vi "SOMD.vi"(8 "Stopp":bool, 10 "SLOT":i32=100, 11 "USB":i32) -> ()   [LabVIEW 2020]
doc: "This VI provides a GUI for SOM-D modules. It implements an abstract module interface, where callers provide the only necessary and sufficient information for callee modules via the datafields USB, SLOT and Stopp. All module intern information are handled hidden by the module. Thereby, a caller must not \"know\" about such internals."
uses:
  <vilib>/Platform/TimedLoop/XDataNode/timing_clust.ctl
  <vilib>/Platform/TimedLoop/XDataNode/nitl_modes.ctl
  <vilib>/Platform/TimedLoop/XDataNode/wakeup.ctl
  <vilib>/platform/TimedLoop/XDataNode/XDataNode.xnode
  <vilib>/Platform/TimedLoop/XDataNode/XDNodeRunTimeDep.lvlib
panel:
  out "DisableBlend":string
  in  "Delayed Data":T1(array[cluster])
  in  "DelayedData[i]":cluster{"Delayed":bool, "ForcedUndelayed":bool}
  in  "SyncNow":bool
  out "SOMD Status":string
  in  "CombiDat 2":T2={"OutputCombi[i]"=[], "MaskedCombi[i]"=TRUE}
  in  "DelayDat 5":cluster{"CoarseDelay[i]":dbl, "FineDelay[i]":u8} {"CoarseDelay[i]" min=-999999.9 max=999999.9 step=1.0 format="%.1f"; "FineDelay[i]" max=63 step=1}
  in  "DelayDat 3":cluster{"CoarseDelay[i]":dbl, "FineDelay[i]":u8} {"CoarseDelay[i]" min=-999999.9 max=999999.9 step=1.0 format="%.1f"; "FineDelay[i]" max=63 step=1}
  in  "DelayDat 6":cluster{"CoarseDelay[i]":dbl, "FineDelay[i]":u8} {"CoarseDelay[i]" min=-999999.9 max=999999.9 step=1.0 format="%.1f"; "FineDelay[i]" max=63 step=1}
  in  "DelayDat 1":cluster{"CoarseDelay[i]":dbl, "FineDelay[i]":u8} {"CoarseDelay[i]" min=-999999.9 max=999999.9 step=1.0 format="%.1f"; "FineDelay[i]" max=63 step=1}
  in  "CombiDat 8":T2={"OutputCombi[i]"=[], "MaskedCombi[i]"=TRUE}
  in  "CombiDat 7":T2={"OutputCombi[i]"=[], "MaskedCombi[i]"=TRUE}
  in  "CombiDat 4":T2={"OutputCombi[i]"=[], "MaskedCombi[i]"=TRUE}
  out "FreqStable":bool caption="stable"
  out "FreqMeasTimer":u32
  out "ExtTriggrd":bool
  out "Trigger Frequency":u32 caption="Trig. Freq. [Hz]"
  in  "CombiDat 5":T2={"OutputCombi[i]"=[], "MaskedCombi[i]"=TRUE}
  in  "CombiDat 3":T2={"OutputCombi[i]"=[], "MaskedCombi[i]"=TRUE}
  in  "DelayDat 8":cluster{"CoarseDelay[i]":dbl, "FineDelay[i]":u8} {"CoarseDelay[i]" min=-999999.9 max=999999.9 step=1.0 format="%.1f"; "FineDelay[i]" max=63 step=1}
  in  "DelayDat 7":cluster{"CoarseDelay[i]":dbl, "FineDelay[i]":u8} {"CoarseDelay[i]" min=-999999.9 max=999999.9 step=1.0 format="%.1f"; "FineDelay[i]" max=63 step=1}
  in  "DelayDat 4":cluster{"CoarseDelay[i]":dbl, "FineDelay[i]":u8} {"CoarseDelay[i]" min=-999999.9 max=999999.9 step=1.0 format="%.1f"; "FineDelay[i]" max=63 step=1}
  in  "CombiDat 6":T2={"OutputCombi[i]"=[], "MaskedCombi[i]"=TRUE}
  in  "CombiDat 1":T2={"OutputCombi[i]"=[], "MaskedCombi[i]"=TRUE}
  in  "Delay Data":T3(array[cluster]) {"CoarseDelay[i]" min=-999999.9 max=999999.9 step=1.0 format="%.1f"; "FineDelay[i]" max=63 step=1}
  in  "DelayDat[i]":cluster{"CoarseDelay[i]":dbl, "FineDelay[i]":u8} {"CoarseDelay[i]" min=-999999.9 max=999999.9 step=1.0 format="%.1f"; "FineDelay[i]" max=63 step=1}
  in  "CombiDat[i]":T2={"OutputCombi[i]"=[], "MaskedCombi[i]"=TRUE}
  in  "Combi Data":T4(array[cluster])
  in  "OutputCombi[i]":bool[](array[boolean])
  in  "Coarse Delay":dbl[](array[numeric])=[1.0, 0.0, 2.0, 0.0, 0.0, 0.0, 0.0, 0.0] min=-999999.9 max=999999.9 format="%.1f"
  in  "Fine Delay":u8[](array[numeric])=[1, 0, 2, 0, 0, 0, 0, 0] max=63 step=1
  in  "BurstDat[i]":T5={"[i]"=1, "BurstLen[i]"=1, "SyncEna[i]"=TRUE, "OutpEna[i]"=TRUE, "Delayed[i]"=TRUE} {"BurstLen[i]" min=0 max=16777215 step=1}
  in  "Burst Data":T6(array[cluster]) {"BurstLen[i]" min=0 max=16777215 step=1}
  in  "AUX In Ctrl":u8(ring) items=["free running", "running if AUX IN is on High", "running if AUX IN is on Low", "disabled"]
  in  "AUX Out Ctrl":u8(ring) items=["disabled", "enabled"]
  in  "Synchronize":bool
  in  "Sync Enable":bool[](array[boolean])=[TRUE, FALSE, FALSE, TRUE, FALSE, FALSE, FALSE, FALSE]
  in  "Burst Out":bool[](array[boolean])=[TRUE, TRUE, FALSE, FALSE, TRUE, FALSE, FALSE, FALSE]
  in  "TriggerLevel [mV]":i32=421 caption="Trig. Level [mV]" min=-1200 max=1200 step=100 format="%5d"
  in  "Burst Length":i32[](array[numeric])=[1, 0, 2, 0, 0, 0, 0, 0]
  in  "Invert":bool=TRUE
  in  "Syncmask":u8
  in  "Presync":u8=4
  in  "Divider":u16=80 min=1 step=1
  in  "Base Osc./Trigger":i32(ring)=2 items=["rising  edge (ext.)", "falling edge (ext.)", "80.00 MHz (int. A)", "64.00 MHz (int. B)", "50.00 MHz (int. C)"]
  in  "DelayDat 2":cluster{"CoarseDelay[i]":dbl, "FineDelay[i]":u8} {"CoarseDelay[i]" min=-999999.9 max=999999.9 step=1.0 format="%.1f"; "FineDelay[i]" max=63 step=1}
  # "Idx   Burst Length       Sync Ena   Out Ena   Delayed"
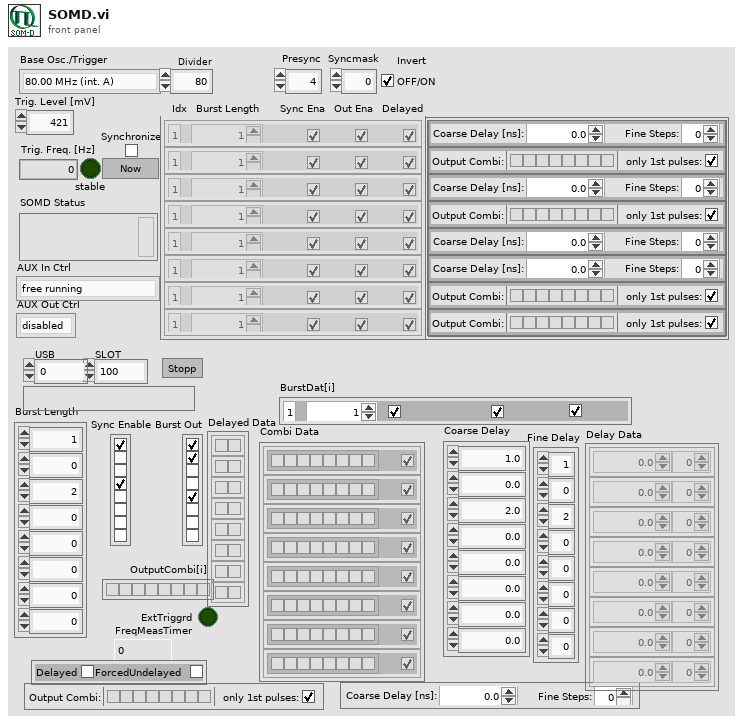
[diagram p1: front panel]
types:
  T1 = cluster{"Delayed":bool, "ForcedUndelayed":bool}[]
  T2 = cluster{"OutputCombi[i]":bool[], "MaskedCombi[i]":bool}
  T3 = cluster{"CoarseDelay[i]":dbl, "FineDelay[i]":u8}[]
  T4 = cluster{"OutputCombi[i]":bool[], "MaskedCombi[i]":bool}[]
  T5 = cluster{"[i]":i32, "BurstLen[i]":i32, "SyncEna[i]":bool, "OutpEna[i]":bool, "Delayed[i]":bool}
  T6 = cluster{"[i]":i32, "BurstLen[i]":i32, "SyncEna[i]":bool, "OutpEna[i]":bool, "Delayed[i]":bool}[]
  T7 = typedef "XDNodeRunTimeDep.lvlib/timing_clust.ctl" = cluster{"Expected End [f-1]":u64, "Actual End [f-1]":u64, "Finished Late? [f-1]":bool, "Expected End [i-1]":u64, "Actual End [i-1]":u64, "Finished Late? [i-1]":bool, "Expected Start [i]":u64, "Actual Start [i]":u64, "Expected Start [f]":u64, "Actual Start [f]":u64, "Source Name":string, "Structure Name":string, "Period":i64, "Deadline":i64, "Offset":i64, "Start":i64, "Priority":i32, "Timeout":i32, "Mode":T8, "Wakeup Reason":T9, "Error":errorcluster, "Source Type":string, "Secondary Source Type":string, "Global End Time":u64, "Global Start Time":u64, "Frame Duration":u64, "Iteration Duration":u64, "Assigned CPU":i32, "I/O Scan Engine Mode":u32}
  T8 = typedef "XDNodeRunTimeDep.lvlib/nitl_modes.ctl" = enum32{"No Change", "Process missed periods, maintain original phase", "Discard missed periods, maintain original phase", "Process missed periods, ignore original phase", "Discard missed periods, ignore original phase"}
  T9 = typedef "XDNodeRunTimeDep.lvlib/wakeup.ctl" = enum32{"Normal", "Aborted", "Asynchronous wakeup", "Timing source error", "Timed loop error", "Timeout"}
  T10 = cluster{"Divider":u16, "PreSync":u8, "SyncMask":u8}
  T11 = cluster{"OutEnable":u8, "SyncEnable":u8, "SyncInverse":enum8{"Standard_Sync_Mask", "Inverse_Sync_Mask"}}
  T12 = typedef "LVPositionTypeDef.ctl" = cluster{"Left":i32, "Top":i32}
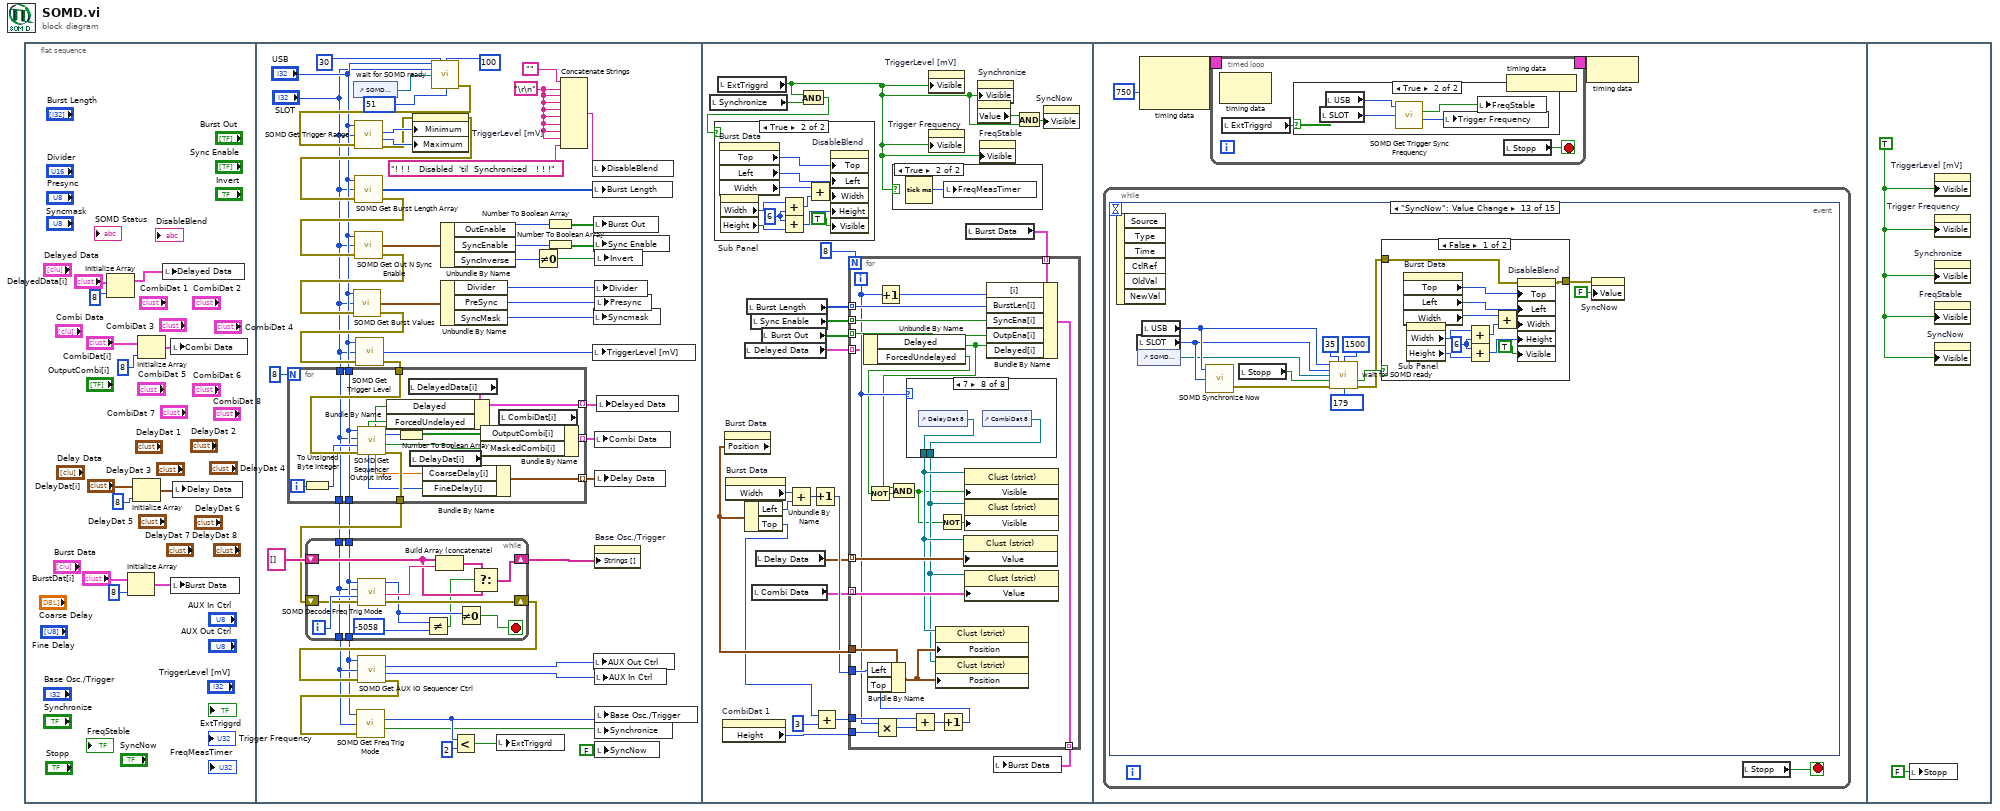
[diagram p0: block diagram]
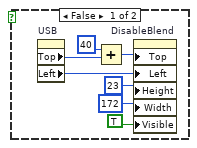
[diagram p2: hidden frame]
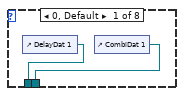
[diagram p4: hidden frame]
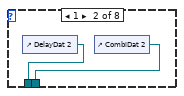
[diagram p5: hidden frame]
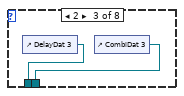
[diagram p6: hidden frame]
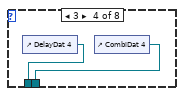
[diagram p7: hidden frame]
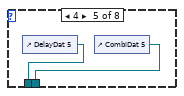
[diagram p8: hidden frame]
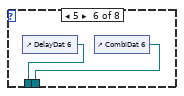
[diagram p9: hidden frame]
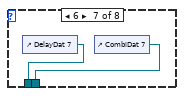
[diagram p10: hidden frame]
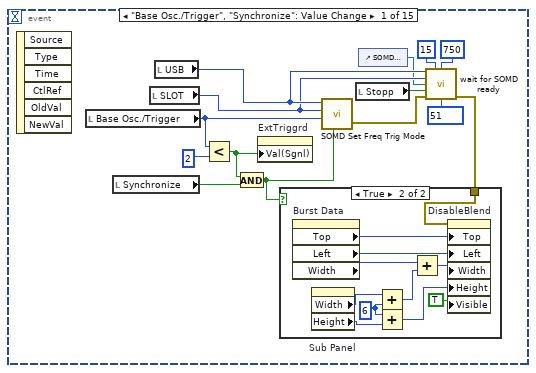
[diagram p12: hidden frame]
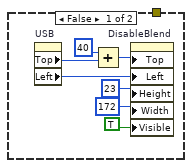
[diagram p13: hidden frame]
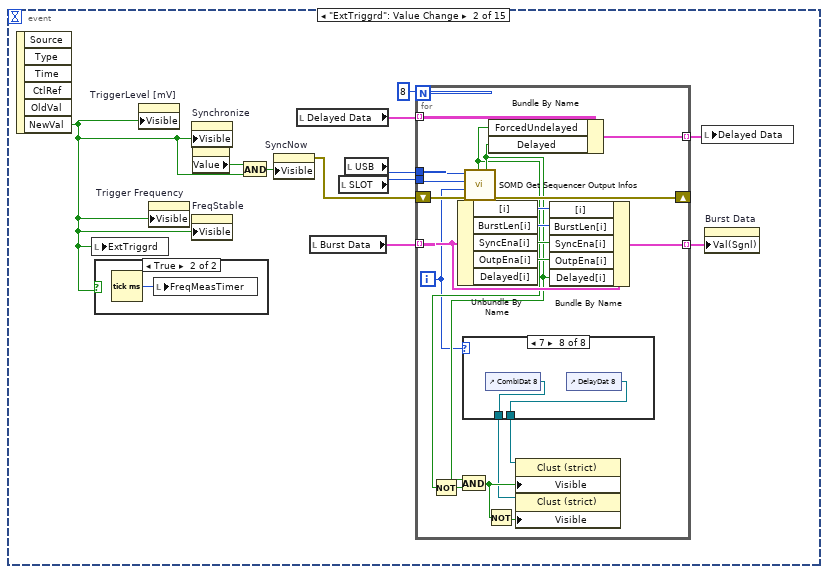
[diagram p14: hidden frame]
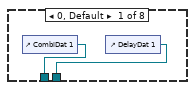
[diagram p15: hidden frame]
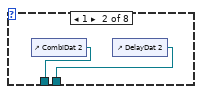
[diagram p16: hidden frame]
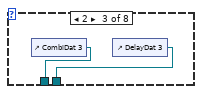
[diagram p17: hidden frame]
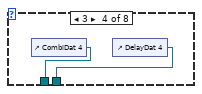
[diagram p18: hidden frame]
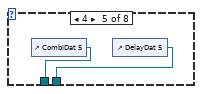
[diagram p19: hidden frame]
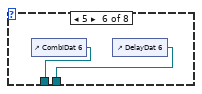
[diagram p20: hidden frame]
diagram:
  n1 = flat-sequence {
    frame #0 {
      n2 = Initialize Array("DelayedData[i]", 8 ("dimension size")) -> (w1:T1)
      n3 = Initialize Array("BurstDat[i]", 8 ("dimension size")) -> (w10:T6)
      n4 = Initialize Array("DelayDat[i]", 8 ("dimension size")) -> (w4:T3)
      n5 = Initialize Array("CombiDat[i]", 8 ("dimension size")) -> (w7:T4)
      n6 = local write "Delayed Data"(w1) -> ()
      n7 = local write "Combi Data"(w7) -> ()
      n8 = local write "Burst Data"(w10) -> ()
      n9 = local write "Delay Data"(w4) -> ()
    }
    frame #1 {
      w13 = "\r\n"
      n10 = control-ref of="SOMD Status"() -> (w21:refnum<vi>)
      n11 = call "wait for SOMD ready.vi"("USB"="USB", "WaitTime"=30, "Max Loops"=100, "SLOT"="SLOT", "InpRefToOutput"=w21, "State Check Mask"=u16 51) -> ("error out"=w24:errorcluster)  [unwired: 5 in, 4 out]
      n12 = call "SOMD Get Trigger Range.vi"("DevIdx"="USB", "SlotId"="SLOT", "error in (no error)"=w24) -> ("MilliVoltLow"=w64:i32, "MilliVoltHigh"=w63:i32, "error out"=w62:errorcluster)  [unwired: 1 out]
      n13 = property on="TriggerLevel [mV]" class="DigNum (strict)"(error in=w62, "Minimum"=w64, "Maximum"=w63) -> (error out=w61:errorcluster)  [unwired: 1 in, 1 out]
      n14 = call "SOMD Get Burst Length Array.vi"("error in (no error)"=w61, "SlotId"="SLOT", "DevIdx"="USB") -> ("error out"=w59:errorcluster, "SOMD Burst Length Array"=w60:i32[])  [unwired: 1 out]
      n15 = call "SOMD Get Out N Sync Enable.vi"("error in (no error)"=w59, "SlotId"="SLOT", "DevIdx"="USB") -> ("error out"=w40:errorcluster, "SOMD Out N Sync Enable"=w58:T11)  [unwired: 1 out]
      n16 = call "SOMD Get Burst Values.vi"("error in (no error)"=w40, "SlotId"="SLOT", "DevIdx"="USB") -> ("error out"=w42:errorcluster, "SOMD Burst Values"=w41:T10)  [unwired: 1 out]
      n17 = call "SOMD Get Trigger Level.vi"("error in (no error)"=w42, "SlotId"="SLOT", "DevIdx"="USB") -> ("error out"=w33:errorcluster, "MilliVolt"=w48:i32)  [unwired: 1 out]
      n18 = for {
        N: 8 -> [_]
        tunnel: [w82] -> w34
        tunnel: w33 -> [w81]
        tunnel: "USB" -> [w79]
        tunnel: [w79] -> w32
        tunnel: "SLOT" -> [w78]
        tunnel: [w78] -> w31
        tunnel: [w66] -> w30 mode=indexing
        tunnel: [w69] -> w29 mode=indexing
        tunnel: [w73] -> w28 mode=indexing
        i -> [w83]
        n19 = To Unsigned Byte Integer(number=w83) -> (unsigned 8bit integer=w80:u8)
        n20 = call "SOMD Get Sequencer Output Infos.vi"("error in (no error)"=w81, "SeqOutputIdx"=w80, "SlotId"=w78, "DevIdx"=w79) -> ("error out"=w82:errorcluster, "Masked Combi"=w74:bool, "bOutputCombi"=w76:u8, "Coarse Delay"=w71:dbl, "Delayed"=w67:bool, "Fine Delay"=w70:u8, "ForcedUndelayed"=w68:bool)  [unwired: 1 out]
        n21 = Number To Boolean Array(number=w76) -> (Boolean array=w75:bool[])
        n22 = local read "DelayedData[i]"() -> (w65:cluster{"Delayed":bool, "ForcedUndelayed":bool})
        n23 = Bundle By Name(cluster=w65, "Delayed"=w67, "ForcedUndelayed"=w68) -> (w66:cluster{"Delayed":bool, "ForcedUndelayed":bool})
        n24 = local read "DelayDat[i]"() -> (w72:cluster{"CoarseDelay[i]":dbl, "FineDelay[i]":u8})
        n25 = Bundle By Name(cluster=w72, "CoarseDelay[i]"=w71, "FineDelay[i]"=w70) -> (w69:cluster{"CoarseDelay[i]":dbl, "FineDelay[i]":u8})
        n26 = local read "CombiDat[i]"() -> (w77:T2)
        n27 = Bundle By Name(cluster=w77, "OutputCombi[i]"=w75, "MaskedCombi[i]"=w74) -> (w73:T2)
      }
      n28 = while {
        tunnel: w32 -> [w85]
        tunnel: w31 -> [w84]
        shift-right: [w94] -> w39
        shift-left: w34 -> [w93]
        shift-right: [w89] -> w46
        shift-left: string[] [] -> [w87]
        tunnel: [w85] -> w25
        tunnel: [w84] -> w26
        i -> [w96]
        stop <- w95 stop-if-true
        n29 = call "SOMD Decode Freq Trig Mode.vi"("error in (no error)"=w93, "FreqTrigMode"=w96, "SlotId"=w84, "DevIdx"=w85) -> ("error out"=w94:errorcluster, "FreqTrigMode"=w92:string, "function return"=w91:i32)
        n30 = Not Equal?(x=w91, y=-5058) -> (x != y?=w86:bool)
        n31 = Build Array (concatenate)(w87, w92) -> (w88:string[])
        n32 = Not Equal To 0?(x=w91) -> (x != 0?=w95:bool)
        n33 = Select(t=w88, s=w86, f=w87) -> (s? t:f=w89:string[])
      }
      n34 = call "SOMD Get AUX IO Sequencer Ctrl.vi"("DevIdx"=w25, "SlotId"=w26, "error in (no error)"=w39) -> ("AUX Out Ctrl"=w37:u8, "AUX In Ctrl"=w36:u8, "error out"=w38:errorcluster)  [unwired: 1 out]
      n35 = call "SOMD Get Freq Trig Mode.vi"("DevIdx"=w25, "SlotId"=w26, "error in (no error)"=w38) -> ("FreqTrigMode"=w45:i32, "Synchronize"=w43:bool)  [unwired: 2 out]
      n36 = Unbundle By Name(w58) -> ("OutEnable"=w57:u8, "SyncEnable"=w55:u8, "SyncInverse"=w53:enum8{"Standard_Sync_Mask", "Inverse_Sync_Mask"})
      n37 = Unbundle By Name(w41) -> ("Divider"=w49:u16, "PreSync"=w50:u8, "SyncMask"=w51:u8)
      n38 = Less?(x=w45, y=2) -> (x < y?=w27:bool)
      n39 = local write "ExtTriggrd"(w27) -> ()
      n40 = Not Equal To 0?(x=w53) -> (x != 0?=w52:bool)
      n41 = Number To Boolean Array(number=w57) -> (Boolean array=w56:bool[])
      n42 = Number To Boolean Array(number=w55) -> (Boolean array=w54:bool[])
      n43 = Concatenate Strings("", w13, w13, w13, w13, w13, w13, w13, w13, "! ! !   Disabled  'til  Synchronized   ! ! !") -> (w16:string)
      n44 = local write "DisableBlend"(w16) -> ()
      n45 = local write "Burst Length"(w60) -> ()
      n46 = local write "TriggerLevel [mV]"(w48) -> ()
      n47 = local write "Burst Out"(w56) -> ()
      n48 = local write "Sync Enable"(w54) -> ()
      n49 = local write "Syncmask"(w51) -> ()
      n50 = local write "AUX Out Ctrl"(w37) -> ()
      n51 = local write "Divider"(w49) -> ()
      n52 = local write "Combi Data"(w28) -> ()
      n53 = local write "AUX In Ctrl"(w36) -> ()
      n54 = local write "Invert"(w52) -> ()
      n55 = local write "Presync"(w50) -> ()
      n56 = local write "Delay Data"(w29) -> ()
      n57 = property on="Base Osc./Trigger" class="Ring (strict)"("Strings []"=w46) -> ()  [unwired: 2 in, 2 out]
      n58 = local write "Base Osc./Trigger"(w45) -> ()
      n59 = local write "Synchronize"(w43) -> ()
      n60 = local write "SyncNow"(FALSE) -> ()
      n61 = local write "Delayed Data"(w30) -> ()
    }
    frame #2 {
      n62 = local read "Synchronize"() -> (w99:bool)
      n63 = local read "ExtTriggrd"() -> (w98:bool)
      n64 = property on="CombiDat 1" class="Clust (strict)"() -> ("Height"=w111:u32)  [unwired: 2 in, 2 out]
      n65 = property on="Burst Data" class="Arr (strict)"() -> ("Position"=w110:T12)  [unwired: 2 in, 2 out]
      n66 = property on="Burst Data" class="Arr (strict)"() -> ("Width"=w109:u32)  [unwired: 2 in, 2 out]
      n67 = local read "Delayed Data"() -> (w113:T1)
      n68 = Unbundle By Name(w110) -> ("Left"=w112:i32, "Top"=w103:i32)
      n69 = local read "Burst Length"() -> (w116:i32[])
      n70 = local read "Sync Enable"() -> (w115:bool[])
      n71 = local read "Combi Data"() -> (w105:T4)
      n72 = local read "Delay Data"() -> (w106:T3)
      n73 = local read "Burst Out"() -> (w114:bool[])
      n74 = Add(x=w109, y=w112) -> (x+y=w107:u32)
      n75 = And(x=w98, y=w99) -> (x .and. y?=w97:bool)
      n76 = case shown="True" w97 {
        frame False {
          n77 = property on="USB" class="DigNum (strict)"() -> ("Top"=w122:i32, "Left"=w126:i32)  [unwired: 2 in, 2 out]
          n78 = Add(x=40, y=w122) -> (x+y=w123:i32)
          n79 = property on="DisableBlend" class="Str"("Top"=w123, "Left"=w126, "Height"=u32 23, "Width"=u32 172 ("Size:Width"), "Visible"=TRUE) -> ()  [unwired: 2 in, 2 out]
        }
        frame True {
          w127 = 6
          n80 = property on="Burst Data" class="Arr (strict)"() -> ("Top"=w136:i32, "Left"=w135:i32, "Width"=w132:u32)  [unwired: 2 in, 2 out]
          n81 = property on="Sub Panel" class="SubPnl"() -> ("Width"=w128:u32, "Height"=w129:u32)  [unwired: 2 in, 2 out]
          n82 = Add(x=w128, y=w127) -> (x+y=w130:u32)
          n83 = Add(x=w127, y=w129) -> (x+y=w131:u32)
          n84 = Add(x=w132, y=w130) -> (x+y=w133:u32)
          n85 = property on="DisableBlend" class="Str"("Top"=w136, "Left"=w135, "Width"=w133, "Height"=w131, "Visible"=TRUE) -> ()  [unwired: 2 in, 2 out]
        }
      }
      n86 = Increment(x=w107) -> (x+1=w108:u32)
      n87 = Add(x=w103, y=3) -> (x+y=w104:i32)
      n88 = case shown="True" w98 {
        frame False {
        }
        frame True {
          n89 = Tick Count (ms)() -> (millisecond timer value=w137:u32)
          n90 = local write "FreqMeasTimer"(w137) -> ()
        }
      }
      n91 = property on="TriggerLevel [mV]" class="DigNum (strict)"("Visible"=w98) -> ()  [unwired: 2 in, 2 out]
      n92 = property on="Trigger Frequency" class="DigNum (strict)"("Visible"=w98) -> ()  [unwired: 2 in, 2 out]
      n93 = local read "Burst Data"() -> (w117:T6)
      n94 = for {
        N: 8 -> [_]
        tunnel: [w161] -> w118 mode=indexing
        tunnel: w117 -> [w162] mode=indexing
        tunnel: w116 -> [w160] mode=indexing
        tunnel: w115 -> [w159] mode=indexing
        tunnel: w114 -> [w158] mode=indexing
        tunnel: w113 -> [w142] mode=indexing
        tunnel: w110 -> [w150]
        tunnel: w111 -> [w156]
        tunnel: w104 -> [w152]
        tunnel: w108 -> [w151]
        tunnel: w106 -> [w147] mode=indexing
        tunnel: w105 -> [w146] mode=indexing
        i -> [w145]
        n95 = Unbundle By Name(w142) -> ("Delayed"=w140:bool, "ForcedUndelayed"=w138:bool)
        n96 = Not(x=w138) -> (.not. x?=w139:bool)
        n97 = Multiply(x=w145, y=w156) -> (x*y=w155:u32)
        n98 = Increment(x=w145) -> (x+1=w157:i32)
        n99 = And(x=w140, y=w139) -> (x .and. y?=w141:bool)
        n100 = case shown="7" w145 {
          tunnel: [w164 w166 w168 w170 w172 w174 w176 w178] -> w144
          tunnel: [w163 w165 w167 w169 w171 w173 w175 w177] -> w143
          frame 0, Default {
            n101 = control-ref of="DelayDat 1"() -> (w164:refnum<vi>)
            n102 = control-ref of="CombiDat 1"() -> (w163:refnum<vi>)
          }
          frame 1 {
            n103 = control-ref of="DelayDat 2"() -> (w166:refnum<vi>)
            n104 = control-ref of="CombiDat 2"() -> (w165:refnum<vi>)
          }
          frame 2 {
            n105 = control-ref of="DelayDat 3"() -> (w168:refnum<vi>)
            n106 = control-ref of="CombiDat 3"() -> (w167:refnum<vi>)
          }
          frame 3 {
            n107 = control-ref of="DelayDat 4"() -> (w170:refnum<vi>)
            n108 = control-ref of="CombiDat 4"() -> (w169:refnum<vi>)
          }
          frame 4 {
            n109 = control-ref of="DelayDat 5"() -> (w172:refnum<vi>)
            n110 = control-ref of="CombiDat 5"() -> (w171:refnum<vi>)
          }
          frame 5 {
            n111 = control-ref of="DelayDat 6"() -> (w174:refnum<vi>)
            n112 = control-ref of="CombiDat 6"() -> (w173:refnum<vi>)
          }
          frame 6 {
            n113 = control-ref of="DelayDat 7"() -> (w176:refnum<vi>)
            n114 = control-ref of="CombiDat 7"() -> (w175:refnum<vi>)
          }
          frame 7 {
            n115 = control-ref of="DelayDat 8"() -> (w178:refnum<vi>)
            n116 = control-ref of="CombiDat 8"() -> (w177:refnum<vi>)
          }
        }
        n117 = Add(x=w152, y=w155) -> (x+y=w154:u32)
        n118 = Not(x=w141) -> (.not. x?=w149:bool)
        n119 = Increment(x=w154) -> (x+1=w153:u32)
        n120 = Bundle By Name(cluster=w150, "Left"=w151, "Top"=w153) -> (w148:T12)
        n121 = property class="Clust (strict)"(reference=w144, "Position"=w148) -> ()  [unwired: 1 in, 2 out]
        n122 = property class="Clust (strict)"(reference=w143, "Position"=w148) -> ()  [unwired: 1 in, 2 out]
        n123 = property class="Clust (strict)"(reference=w144, "Value"=w147) -> ()  [unwired: 1 in, 2 out]
        n124 = property class="Clust (strict)"(reference=w144, "Visible"=w141) -> ()  [unwired: 1 in, 2 out]
        n125 = property class="Clust (strict)"(reference=w143, "Visible"=w149) -> ()  [unwired: 1 in, 2 out]
        n126 = property class="Clust (strict)"(reference=w143, "Value"=w146) -> ()  [unwired: 1 in, 2 out]
        n127 = Bundle By Name(cluster=w162, "[i]"=w157, "BurstLen[i]"=w160, "SyncEna[i]"=w159, "OutpEna[i]"=w158, "Delayed[i]"=w140) -> (w161:T5)
      }
      n128 = property on="Synchronize" class="Bool (strict)"("Visible"=w98) -> ()  [unwired: 2 in, 2 out]
      n129 = property on="Synchronize" class="Bool (strict)"() -> ("Value"=w100:bool)  [unwired: 2 in, 2 out]
      n130 = property on="FreqStable" class="Bool (strict)"("Visible"=w98) -> ()  [unwired: 2 in, 2 out]
      n131 = local write "Burst Data"(w118) -> ()
      n132 = And(x=w100, y=w98) -> (x .and. y?=w101:bool)
      n133 = property on="SyncNow" class="Bool (strict)"("Visible"=w101) -> ()  [unwired: 2 in, 2 out]
    }
    frame #3 {
      n134 = while {
        stop <- w194 stop-if-true
        n135 = event shown="[12] \"SyncNow\": Value Change" {
          selector: _ -> [_ _ _ _ _ _ _ _ _ _ _ _ _ _ _]
          dyn-events: _ -> [_ _ _ _ _ _ _ _ _ _ _ _ _ _ _]
          timeout: _ -> [_ _ _ _ _ _ _ _ _ _ _ _ _ _ _]
          event "Base Osc./Trigger", "Synchronize": Value Change {
            n136 = event-data() -> ()  [unwired: 1 in, 6 out]
            n137 = local read "Base Osc./Trigger"() -> (w207:i32)
            n138 = local read "Synchronize"() -> (w197:bool)
            n139 = local read "SLOT"() -> (w202:i32)
            n140 = local read "USB"() -> (w203:i32)
            n141 = Less?(x=w207, y=2) -> (x < y?=w198:bool)
            n142 = And(x=w198, y=w197) -> (x .and. y?=w196:bool)
            n143 = property on="ExtTriggrd" class="Bool (strict)"("Val(Sgnl)"=w198) -> ()  [unwired: 2 in, 2 out]
            n144 = call "SOMD Set Freq Trig Mode.vi"("DevIdx"=w203, "SlotId"=w202, "FreqTrigMode"=w207, "Synchronize"=w196) -> ("error out"=w206:errorcluster)  [unwired: 1 in, 1 out]
            n145 = local read "Stopp"() -> (w200:bool)
            n146 = control-ref of="SOMD Status"() -> (w201:refnum<vi>)
            n147 = call "wait for SOMD ready.vi"("USB"=w203, "WaitTime"=15, "Max Loops"=750, "SLOT"=w202, "InpRefToOutput"=w201, "Stopp"=w200, "error in (no error)"=w206, "State Check Mask"=u16 51) -> ("error out"=w195:errorcluster)  [unwired: 3 in, 4 out]
            n148 = case shown="True" w196 {
              tunnel: w195 -> [_ w216]
              frame False {
                n149 = property on="USB" class="DigNum (strict)"() -> ("Top"=w211:i32, "Left"=w215:i32)  [unwired: 2 in, 2 out]
                n150 = Add(x=40, y=w211) -> (x+y=w212:i32)
                n151 = property on="DisableBlend" class="Str"("Top"=w212, "Left"=w215, "Height"=u32 23, "Width"=u32 172 ("Size:Width"), "Visible"=TRUE) -> ()  [unwired: 2 in, 2 out]
              }
              frame True {
                w220 = 6
                n152 = property on="Burst Data" class="Arr (strict)"() -> ("Top"=w226:i32, "Left"=w225:i32, "Width"=w222:u32)  [unwired: 2 in, 2 out]
                n153 = property on="Sub Panel" class="SubPnl"() -> ("Width"=w218:u32, "Height"=w219:u32)  [unwired: 2 in, 2 out]
                n154 = Add(x=w218, y=w220) -> (x+y=w217:u32)
                n155 = Add(x=w220, y=w219) -> (x+y=w221:u32)
                n156 = Add(x=w222, y=w217) -> (x+y=w223:u32)
                n157 = property on="DisableBlend" class="Str"(error in=w216, "Top"=w226, "Left"=w225, "Width"=w223, "Height"=w221, "Visible"=TRUE) -> ()  [unwired: 1 in, 2 out]
              }
            }
          }
          event "ExtTriggrd": Value Change {
            n158 = event-data() -> ("NewVal"=w235:bool)  [unwired: 1 in, 5 out]
            n159 = local write "ExtTriggrd"(w235) -> ()
            n160 = case shown="True" w235 {
              frame False {
              }
              frame True {
                n161 = Tick Count (ms)() -> (millisecond timer value=w274:u32)
                n162 = local write "FreqMeasTimer"(w274) -> ()
              }
            }
            n163 = property on="TriggerLevel [mV]" class="DigNum (strict)"("Visible"=w235) -> ()  [unwired: 2 in, 2 out]
            n164 = property on="Trigger Frequency" class="DigNum (strict)"("Visible"=w235) -> ()  [unwired: 2 in, 2 out]
            n165 = property on="Synchronize" class="Bool (strict)"("Visible"=w235) -> ()  [unwired: 2 in, 2 out]
            n166 = property on="FreqStable" class="Bool (strict)"("Visible"=w235) -> ()  [unwired: 2 in, 2 out]
            n167 = property on="Synchronize" class="Bool (strict)"() -> ("Value"=w236:bool)  [unwired: 2 in, 2 out]
            n168 = And(x=w236, y=w235) -> (x .and. y?=w237:bool)
            n169 = property on="SyncNow" class="Bool (strict)"("Visible"=w237) -> (error out=w228:errorcluster)  [unwired: 2 in, 1 out]
            n170 = local read "Delayed Data"() -> (w231:T1)
            n171 = local read "Burst Data"() -> (w229:T6)
            n172 = local read "SLOT"() -> (w232:i32)
            n173 = local read "USB"() -> (w233:i32)
            n174 = for {
              N: 8 -> [_]
              shift-right: [w257] -> _
              shift-left: w228 -> [w256]
              tunnel: w233 -> [w255]
              tunnel: w232 -> [w254]
              tunnel: w231 -> [w253] mode=indexing
              tunnel: [w252] -> w230 mode=indexing
              tunnel: w229 -> [w251] mode=indexing
              tunnel: [w246] -> w227 mode=indexing
              i -> [w240]
              n175 = Unbundle By Name(w251) -> ("[i]"=w247:i32, "BurstLen[i]"=w248:i32, "SyncEna[i]"=w249:bool, "OutpEna[i]"=w250:bool)  [unwired: 1 out]
              n176 = case shown="7" w240 {
                tunnel: [w259 w260 w262 w264 w266 w268 w270 w272] -> w239
                tunnel: [w258 w261 w263 w265 w267 w269 w271 w273] -> w238
                frame 0, Default {
                  n177 = control-ref of="CombiDat 1"() -> (w258:refnum<vi>)
                  n178 = control-ref of="DelayDat 1"() -> (w259:refnum<vi>)
                }
                frame 1 {
                  n179 = control-ref of="CombiDat 2"() -> (w261:refnum<vi>)
                  n180 = control-ref of="DelayDat 2"() -> (w260:refnum<vi>)
                }
                frame 2 {
                  n181 = control-ref of="CombiDat 3"() -> (w263:refnum<vi>)
                  n182 = control-ref of="DelayDat 3"() -> (w262:refnum<vi>)
                }
                frame 3 {
                  n183 = control-ref of="CombiDat 4"() -> (w265:refnum<vi>)
                  n184 = control-ref of="DelayDat 4"() -> (w264:refnum<vi>)
                }
                frame 4 {
                  n185 = control-ref of="CombiDat 5"() -> (w267:refnum<vi>)
                  n186 = control-ref of="DelayDat 5"() -> (w266:refnum<vi>)
                }
                frame 5 {
                  n187 = control-ref of="CombiDat 6"() -> (w269:refnum<vi>)
                  n188 = control-ref of="DelayDat 6"() -> (w268:refnum<vi>)
                }
                frame 6 {
                  n189 = control-ref of="CombiDat 7"() -> (w271:refnum<vi>)
                  n190 = control-ref of="DelayDat 7"() -> (w270:refnum<vi>)
                }
                frame 7 {
                  n191 = control-ref of="CombiDat 8"() -> (w273:refnum<vi>)
                  n192 = control-ref of="DelayDat 8"() -> (w272:refnum<vi>)
                }
              }
              n193 = call "SOMD Get Sequencer Output Infos.vi"("error in (no error)"=w256, "SeqOutputIdx"=w240, "SlotId"=w254, "DevIdx"=w255) -> ("error out"=w257:errorcluster, "Delayed"=w242:bool, "ForcedUndelayed"=w241:bool)  [unwired: 5 out]
              n194 = Not(x=w241) -> (.not. x?=w245:bool)
              n195 = And(x=w242, y=w245) -> (x .and. y?=w243:bool)
              n196 = Not(x=w243) -> (.not. x?=w244:bool)
              n197 = Bundle By Name(cluster=w253, "ForcedUndelayed"=w241, "Delayed"=w242) -> (w252:cluster{"Delayed":bool, "ForcedUndelayed":bool})
              n198 = property class="Clust (strict)"(reference=w239, "Visible"=w243) -> ()  [unwired: 1 in, 2 out]
              n199 = property class="Clust (strict)"(reference=w238, "Visible"=w244) -> ()  [unwired: 1 in, 2 out]
              n200 = Bundle By Name(cluster=w251, "[i]"=w247, "BurstLen[i]"=w248, "SyncEna[i]"=w249, "OutpEna[i]"=w250, "Delayed[i]"=w242) -> (w246:T5)
            }
            n201 = local write "Delayed Data"(w230) -> ()
            n202 = property on="Burst Data" class="Arr (strict)"("Val(Sgnl)"=w227) -> ()  [unwired: 2 in, 2 out]
          }
          event "TriggerLevel [mV]": Value Change {
            n203 = event-data() -> ()  [unwired: 1 in, 6 out]
            n204 = local read "TriggerLevel [mV]"() -> (w275:i32)
            n205 = local read "SLOT"() -> (w277:i32)
            n206 = local read "USB"() -> (w276:i32)
            n207 = call "SOMD Set Trigger Level.vi"("MilliVolt"=w275, "SlotId"=w277, "DevIdx"=w276) -> ()  [unwired: 1 in, 2 out]
          }
          event "Divider", "Presync", "Syncmask": Value Change {
            n208 = event-data() -> ()  [unwired: 1 in, 6 out]
            n209 = local read "Syncmask"() -> (w287:u8)
            n210 = local read "Presync"() -> (w288:u8)
            n211 = local read "Divider"() -> (w289:u16)
            n212 = local read "SLOT"() -> (w281:i32)
            n213 = local read "USB"() -> (w282:i32)
            n214 = Bundle By Name(cluster=T10 {"Divider"=0, "PreSync"=0, "SyncMask"=0} ("SOM Burst Values"), "Divider"=w289, "PreSync"=w288, "SyncMask"=w287) -> (w286:T10)
            n215 = call "SOMD Set Burst Values.vi"("SOMD Burst Values"=w286, "SlotId"=w281, "DevIdx"=w282) -> ("error out"=w278:errorcluster)  [unwired: 1 in, 1 out]
            n216 = local read "Stopp"() -> (w279:bool)
            n217 = control-ref of="SOMD Status"() -> (w280:refnum<vi>)
            n218 = call "wait for SOMD ready.vi"("USB"=w282, "WaitTime"=15, "Max Loops"=750, "SLOT"=w281, "InpRefToOutput"=w280, "Stopp"=w279, "error in (no error)"=w278, "State Check Mask"=u16 51) -> ()  [unwired: 3 in, 5 out]
          }
          event "Burst Length": Value Change {
            n219 = event-data() -> ()  [unwired: 1 in, 6 out]
            n220 = local read "Combi Data"() -> (w292:T4)
            n221 = local read "Delay Data"() -> (w291:T3)
            n222 = local read "Delayed Data"() -> (w295:T1)
            n223 = local read "Burst Length"() -> (w298:i32[])
            n224 = local read "Sync Enable"() -> (w293:bool[])
            n225 = local read "Burst Data"() -> (w297:T6)
            n226 = local read "Burst Out"() -> (w294:bool[])
            n227 = local read "SLOT"() -> (w300:i32)
            n228 = local read "USB"() -> (w301:i32)
            n229 = for {
              N: 8 -> [_]
              tunnel: w298 -> [w318] mode=indexing
              tunnel: w293 -> [w317] mode=indexing
              tunnel: w294 -> [w316] mode=indexing
              tunnel: w297 -> [w315] mode=indexing
              tunnel: [w314] -> w296 mode=indexing
              tunnel: w295 -> [w306] mode=indexing
              tunnel: w292 -> [w309] mode=indexing
              tunnel: w291 -> [w310] mode=indexing
              i -> [w312]
              n230 = Increment(x=w312) -> (x+1=w313:i32)
              n231 = Unbundle By Name(w306) -> ("Delayed"=w303:bool, "ForcedUndelayed"=w302:bool)
              n232 = Not(x=w302) -> (.not. x?=w304:bool)
              n233 = And(x=w303, y=w304) -> (x .and. y?=w305:bool)
              n234 = case shown="7" w312 {
                tunnel: [w320 w322 w324 w326 w328 w330 w332 w334] -> w307
                tunnel: [w319 w321 w323 w325 w327 w329 w331 w333] -> w308
                frame 0, Default {
                  n235 = control-ref of="DelayDat 1"() -> (w320:refnum<vi>)
                  n236 = control-ref of="CombiDat 1"() -> (w319:refnum<vi>)
                }
                frame 1 {
                  n237 = control-ref of="DelayDat 2"() -> (w322:refnum<vi>)
                  n238 = control-ref of="CombiDat 2"() -> (w321:refnum<vi>)
                }
                frame 2 {
                  n239 = control-ref of="DelayDat 3"() -> (w324:refnum<vi>)
                  n240 = control-ref of="CombiDat 3"() -> (w323:refnum<vi>)
                }
                frame 3 {
                  n241 = control-ref of="DelayDat 4"() -> (w326:refnum<vi>)
                  n242 = control-ref of="CombiDat 4"() -> (w325:refnum<vi>)
                }
                frame 4 {
                  n243 = control-ref of="DelayDat 5"() -> (w328:refnum<vi>)
                  n244 = control-ref of="CombiDat 5"() -> (w327:refnum<vi>)
                }
                frame 5 {
                  n245 = control-ref of="DelayDat 6"() -> (w330:refnum<vi>)
                  n246 = control-ref of="CombiDat 6"() -> (w329:refnum<vi>)
                }
                frame 6 {
                  n247 = control-ref of="DelayDat 7"() -> (w332:refnum<vi>)
                  n248 = control-ref of="CombiDat 7"() -> (w331:refnum<vi>)
                }
                frame 7 {
                  n249 = control-ref of="DelayDat 8"() -> (w334:refnum<vi>)
                  n250 = control-ref of="CombiDat 8"() -> (w333:refnum<vi>)
                }
              }
              n251 = Not(x=w305) -> (.not. x?=w311:bool)
              n252 = property class="Clust (strict)"(reference=w307, "Value"=w310) -> ()  [unwired: 1 in, 2 out]
              n253 = property class="Clust (strict)"(reference=w307, "Visible"=w305) -> ()  [unwired: 1 in, 2 out]
              n254 = property class="Clust (strict)"(reference=w308, "Visible"=w311) -> ()  [unwired: 1 in, 2 out]
              n255 = property class="Clust (strict)"(reference=w308, "Value"=w309) -> ()  [unwired: 1 in, 2 out]
              n256 = Bundle By Name(cluster=w315, "[i]"=w313, "BurstLen[i]"=w318, "SyncEna[i]"=w317, "OutpEna[i]"=w316, "Delayed[i]"=w303) -> (w314:T5)
            }
            n257 = call "SOMD Set Burst Length Array.vi"("SOMD Burst Length Array"=w298, "SlotId"=w300, "DevIdx"=w301) -> ()  [unwired: 1 in, 2 out]
            n258 = local write "Burst Data"(w296) -> ()
          }
          event "Invert", "Burst Out", "Sync Enable": Value Change {
            n259 = event-data() -> ()  [unwired: 1 in, 6 out]
            n260 = local read "Delayed Data"() -> (w335:T1)
            n261 = local read "Burst Length"() -> (w338:i32[])
            n262 = local read "Sync Enable"() -> (w336:bool[])
            n263 = local read "Burst Data"() -> (w341:T6)
            n264 = local read "Burst Out"() -> (w337:bool[])
            n265 = local read "Invert"() -> (w345:bool)
            n266 = Boolean To (0,1)(Boolean=w345) -> (0, 1=w342:i16)
            n267 = Boolean Array To Number(Boolean array=w336) -> (number=w347:u8)
            n268 = Boolean Array To Number(Boolean array=w337) -> (number=w346:u8)
            n269 = for {
              N: 8 -> [_]
              tunnel: w338 -> [w359] mode=indexing
              tunnel: w336 -> [w358] mode=indexing
              tunnel: w337 -> [w357] mode=indexing
              tunnel: w341 -> [w356] mode=indexing
              tunnel: [w355] -> w340 mode=indexing
              tunnel: w335 -> [w352] mode=indexing
              i -> [w353]
              n270 = Unbundle By Name(w352) -> ("Delayed"=w351:bool)
              n271 = Increment(x=w353) -> (x+1=w354:i32)
              n272 = Bundle By Name(cluster=w356, "[i]"=w354, "BurstLen[i]"=w359, "SyncEna[i]"=w358, "OutpEna[i]"=w357, "Delayed[i]"=w351) -> (w355:T5)
            }
            n273 = To Unsigned Byte Integer(number=w342) -> (unsigned 8bit integer=w343:u8)
            n274 = local read "SLOT"() -> (w350:i32)
            n275 = local read "USB"() -> (w349:i32)
            n276 = Bundle By Name(cluster=T11 {"OutEnable"=0, "SyncEnable"=0, "SyncInverse"=enum."Standard_Sync_Mask"} ("SOM Out N Sync Enable"), "OutEnable"=w346, "SyncEnable"=w347, "SyncInverse"=w343) -> (w344:T11)
            n277 = call "SOMD Set Out N Sync Enable.vi"("SOM Out N Sync Enable"=w344, "SlotId"=w350, "DevIdx"=w349) -> ()  [unwired: 1 in, 2 out]
            n278 = local write "Burst Data"(w340) -> ()
          }
          event "AUX In Ctrl", "AUX Out Ctrl": Value Change {
            n279 = event-data() -> ()  [unwired: 1 in, 6 out]
            n280 = local read "AUX Out Ctrl"() -> (w360:u8)
            n281 = local read "AUX In Ctrl"() -> (w363:u8)
            n282 = local read "SLOT"() -> (w361:i32)
            n283 = local read "USB"() -> (w362:i32)
            n284 = call "SOMD Set AUX IO Sequencer Ctrl.vi"("DevIdx"=w362, "SlotId"=w361, "AUX Out Ctrl"=w360, "AUX In Ctrl"=w363) -> ()  [unwired: 1 in, 2 out]
          }
          event "Burst Data": Value Change {
            n285 = event-data() -> ("OldVal"=w373:T6, "NewVal"=w372:T6)  [unwired: 1 in, 4 out]
            n286 = local read "Combi Data"() -> (w368:T4)
            n287 = local read "Delay Data"() -> (w369:T3)
            n288 = local read "SLOT"() -> (w366:i32)
            n289 = local read "USB"() -> (w367:i32)
            n290 = local read "Delayed Data"() -> (w365:T1)
            n291 = for {
              N: 8 -> [_]
              tunnel: w373 -> [w396] mode=indexing
              tunnel: w372 -> [w395] mode=indexing
              tunnel: [w394] -> w370 mode=indexing
              tunnel: w369 -> [w380] mode=indexing
              tunnel: w368 -> [w379] mode=indexing
              tunnel: w367 -> [w377]
              tunnel: w366 -> [w376]
              tunnel: w365 -> [w375] mode=indexing
              tunnel: [w374] -> w364 mode=indexing
              i -> [w382]
              n292 = Unbundle By Name(w396) -> ("BurstLen[i]"=w392:i32, "SyncEna[i]"=w390:bool, "OutpEna[i]"=w387:bool, "Delayed[i]"=w385:bool)  [unwired: 1 out]
              n293 = Unbundle By Name(w395) -> ("BurstLen[i]"=w391:i32, "SyncEna[i]"=w388:bool, "OutpEna[i]"=w383:bool, "Delayed[i]"=w381:bool)  [unwired: 1 out]
              n294 = Not Equal?(x=w385, y=w381) -> (x != y?=w384:bool)
              n295 = case shown="True" w384 {
                tunnel: w382 -> [_ w407]
                tunnel: w381 -> [_ w417]
                tunnel: w380 -> [_ w415]
                tunnel: w379 -> [_ w412]
                tunnel: w377 -> [_ w409]
                tunnel: w376 -> [_ w408]
                tunnel: w375 -> [w401 w405]
                tunnel: [w401 w404] -> w374
                frame False {
                }
                frame True {
                  n296 = Unbundle By Name(w415) -> ("CoarseDelay[i]"=w414:dbl, "FineDelay[i]"=w413:u8)
                  n297 = Unbundle By Name(w412) -> ("OutputCombi[i]"=w410:bool[], "MaskedCombi[i]"=w411:bool)
                  n298 = call "SOMD Set Sequencer Output Infos.vi"("DevIdx"=w409, "Output Combi"=w410, "Masked Combi"=w411, "SlotId"=w408, "Seq. Output Idx"=w407, "Delayed"=w417, "Coarse Delay"=w414, "Fine Delay"=w413) -> ("error out"=w416:errorcluster)  [unwired: 6 in, 1 out]
                  n299 = Not(x=w417) -> (.not. x?=w425:bool)
                  n300 = case shown="0, Default" w407 {
                    tunnel: [w427 w429 w431 w433 w435 w437 w439 w441] -> w424
                    tunnel: [w426 w428 w430 w432 w434 w436 w438 w440] -> w423
                    frame 0, Default {
                      n301 = control-ref of="DelayDat 1"() -> (w427:refnum<vi>)
                      n302 = control-ref of="CombiDat 1"() -> (w426:refnum<vi>)
                    }
                    frame 1 {
                      n303 = control-ref of="DelayDat 2"() -> (w429:refnum<vi>)
                      n304 = control-ref of="CombiDat 2"() -> (w428:refnum<vi>)
                    }
                    frame 2 {
                      n305 = control-ref of="DelayDat 3"() -> (w431:refnum<vi>)
                      n306 = control-ref of="CombiDat 3"() -> (w430:refnum<vi>)
                    }
                    frame 3 {
                      n307 = control-ref of="DelayDat 4"() -> (w433:refnum<vi>)
                      n308 = control-ref of="CombiDat 4"() -> (w432:refnum<vi>)
                    }
                    frame 4 {
                      n309 = control-ref of="DelayDat 5"() -> (w435:refnum<vi>)
                      n310 = control-ref of="CombiDat 5"() -> (w434:refnum<vi>)
                    }
                    frame 5 {
                      n311 = control-ref of="DelayDat 6"() -> (w437:refnum<vi>)
                      n312 = control-ref of="CombiDat 6"() -> (w436:refnum<vi>)
                    }
                    frame 6 {
                      n313 = control-ref of="DelayDat 7"() -> (w439:refnum<vi>)
                      n314 = control-ref of="CombiDat 7"() -> (w438:refnum<vi>)
                    }
                    frame 7 {
                      n315 = control-ref of="DelayDat 8"() -> (w441:refnum<vi>)
                      n316 = control-ref of="CombiDat 8"() -> (w440:refnum<vi>)
                    }
                  }
                  n317 = property class="Clust (strict)"(reference=w424, "Visible"=w417) -> ()  [unwired: 1 in, 2 out]
                  n318 = property class="Clust (strict)"(reference=w424, "Value"=w415) -> ()  [unwired: 1 in, 2 out]
                  n319 = property class="Clust (strict)"(reference=w423, "Visible"=w425) -> ()  [unwired: 1 in, 2 out]
                  n320 = property class="Clust (strict)"(reference=w423, "Value"=w412) -> ()  [unwired: 1 in, 2 out]
                  n321 = control-ref of="SOMD Status"() -> (w418:refnum<vi>)
                  n322 = local read "Stopp"() -> (w419:bool)
                  n323 = call "wait for SOMD ready.vi"("USB"=w409, "WaitTime"=15, "Max Loops"=750, "SLOT"=w408, "InpRefToOutput"=w418, "Stopp"=w419, "error in (no error)"=w416, "State Check Mask"=u16 51) -> ("error out"=w406:errorcluster)  [unwired: 3 in, 4 out]
                  n324 = call "SOMD Get Sequencer Output Infos.vi"("error in (no error)"=w406, "SeqOutputIdx"=w407, "SlotId"=w408, "DevIdx"=w409) -> ("Delayed"=w403:bool, "ForcedUndelayed"=w402:bool)  [unwired: 6 out]
                  n325 = Bundle By Name(cluster=w405, "Delayed"=w403, "ForcedUndelayed"=w402) -> (w404:cluster{"Delayed":bool, "ForcedUndelayed":bool})
                }
              }
              n326 = Not Equal?(x=w387, y=w383) -> (x != y?=w386:bool)
              n327 = case shown="True" w386 {
                tunnel: w383 -> [_ w399]
                tunnel: w382 -> [_ w398]
                frame False {
                }
                frame True {
                  n328 = local read "Burst Out"() -> (w400:bool[])
                  n329 = Replace Array Subset(array=w400, new element=w399, index=w398) -> (w397:bool[])
                  n330 = property on="Burst Out" class="Arr (strict)"("Val(Sgnl)"=w397) -> ()  [unwired: 2 in, 2 out]
                }
              }
              n331 = Not Equal?(x=w390, y=w388) -> (x != y?=w389:bool)
              n332 = Not Equal?(x=w392, y=w391) -> (x != y?=w393:bool)
              n333 = case shown="True" w393 {
                tunnel: w382 -> [_ w447]
                tunnel: w391 -> [_ w448]
                frame False {
                }
                frame True {
                  n334 = local read "Burst Length"() -> (w449:i32[])
                  n335 = Replace Array Subset(array=w449, new element=w448, index=w447) -> (w446:i32[])
                  n336 = property on="Burst Length" class="Arr (strict)"("Val(Sgnl)"=w446) -> ()  [unwired: 2 in, 2 out]
                }
              }
              n337 = case shown="True" w389 {
                tunnel: w382 -> [_ w444]
                tunnel: w388 -> [_ w443]
                frame False {
                }
                frame True {
                  n338 = local read "Sync Enable"() -> (w445:bool[])
                  n339 = Replace Array Subset(array=w445, new element=w443, index=w444) -> (w442:bool[])
                  n340 = property on="Sync Enable" class="Arr (strict)"("Val(Sgnl)"=w442) -> ()  [unwired: 2 in, 2 out]
                }
              }
              n341 = Increment(x=w382) -> (x+1=w378:i32)
              n342 = Bundle By Name(cluster=w395, "[i]"=w378, "BurstLen[i]"=w391, "SyncEna[i]"=w388, "OutpEna[i]"=w383, "Delayed[i]"=w381) -> (w394:T5)
            }
            n343 = local write "Burst Data"(w370) -> ()
            n344 = local write "Delayed Data"(w364) -> ()
          }
          event "Delay Data": Value Change {
            n345 = event-data() -> ("OldVal"=w453:T3, "NewVal"=w454:T3)  [unwired: 1 in, 4 out]
            n346 = local read "Combi Data"() -> (w450:T4)
            n347 = local read "Burst Data"() -> (w451:T6)
            n348 = for {
              N: 8 -> [_]
              tunnel: w454 -> [w457] mode=indexing
              tunnel: w453 -> [w470] mode=indexing
              tunnel: w451 -> [w459] mode=indexing
              tunnel: w450 -> [w458] mode=indexing
              shift-right: [w455] -> _
              shift-left: _ -> [w456]
              i -> [w462]
              n349 = local read "SLOT"() -> (w461:i32)
              n350 = local read "USB"() -> (w460:i32)
              n351 = Unbundle By Name(w457) -> ("CoarseDelay[i]"=w464:dbl, "FineDelay[i]"=w463:u8)
              n352 = Unbundle By Name(w470) -> ("CoarseDelay[i]"=w466:dbl, "FineDelay[i]"=w467:u8)
              n353 = Not Equal?(x=w466, y=w464) -> (x != y?=w468:bool)
              n354 = Not Equal?(x=w467, y=w463) -> (x != y?=w469:bool)
              n355 = Or(x=w468, y=w469) -> (x .or. y?=w465:bool)
              n356 = case shown="True" w465 {
                tunnel: w459 -> [_ w493]
                tunnel: w462 -> [_ w485]
                tunnel: w461 -> [_ w491]
                tunnel: w460 -> [_ w490]
                tunnel: w464 -> [_ w489]
                tunnel: w463 -> [_ w488]
                tunnel: w458 -> [_ w487]
                tunnel: w457 -> [_ w484]
                tunnel: w456 -> [w471 w483]
                tunnel: [w471 w475] -> w455
                frame False {
                }
                frame True {
                  n357 = Unbundle By Name(w487) -> ("MaskedCombi[i]"=w472:bool, "OutputCombi[i]"=w473:bool[])
                  n358 = case shown="0, Default" w485 {
                    tunnel: w484 -> [w494 w496 w498 w500 w502 w504 w506 w508]
                    frame 0, Default {
                      n359 = control-ref of="DelayDat 1"() -> (w495:refnum<vi>)
                      n360 = property class="Clust (strict)"(reference=w495, "Value"=w494) -> ()  [unwired: 1 in, 2 out]
                    }
                    frame 1 {
                      n361 = control-ref of="DelayDat 2"() -> (w497:refnum<vi>)
                      n362 = property class="Clust (strict)"(reference=w497, "Value"=w496) -> ()  [unwired: 1 in, 2 out]
                    }
                    frame 2 {
                      n363 = control-ref of="DelayDat 3"() -> (w499:refnum<vi>)
                      n364 = property class="Clust (strict)"(reference=w499, "Value"=w498) -> ()  [unwired: 1 in, 2 out]
                    }
                    frame 3 {
                      n365 = control-ref of="DelayDat 4"() -> (w501:refnum<vi>)
                      n366 = property class="Clust (strict)"(reference=w501, "Value"=w500) -> ()  [unwired: 1 in, 2 out]
                    }
                    frame 4 {
                      n367 = control-ref of="DelayDat 5"() -> (w503:refnum<vi>)
                      n368 = property class="Clust (strict)"(reference=w503, "Value"=w502) -> ()  [unwired: 1 in, 2 out]
                    }
                    frame 5 {
                      n369 = control-ref of="DelayDat 6"() -> (w505:refnum<vi>)
                      n370 = property class="Clust (strict)"(reference=w505, "Value"=w504) -> ()  [unwired: 1 in, 2 out]
                    }
                    frame 6 {
                      n371 = control-ref of="DelayDat 7"() -> (w507:refnum<vi>)
                      n372 = property class="Clust (strict)"(reference=w507, "Value"=w506) -> ()  [unwired: 1 in, 2 out]
                    }
                    frame 7 {
                      n373 = control-ref of="DelayDat 8"() -> (w509:refnum<vi>)
                      n374 = property class="Clust (strict)"(reference=w509, "Value"=w508) -> ()  [unwired: 1 in, 2 out]
                    }
                  }
                  n375 = Unbundle By Name(w493) -> ("Delayed[i]"=w492:bool)
                  n376 = To Unsigned Byte Integer(number=w485) -> (unsigned 8bit integer=w486:u8)
                  n377 = call "SOMD Set Sequencer Output Infos.vi"("DevIdx"=w490, "Output Combi"=w473, "Masked Combi"=w472, "SlotId"=w491, "Seq. Output Idx"=w486, "Delayed"=w492, "error in (no error)"=w483, "Coarse Delay"=w489, "Fine Delay"=w488) -> ("error out"=w474:errorcluster)  [unwired: 5 in, 1 out]
                  n378 = local read "Stopp"() -> (w479:bool)
                  n379 = local read "SLOT"() -> (w481:i32)
                  n380 = control-ref of="SOMD Status"() -> (w480:refnum<vi>)
                  n381 = local read "USB"() -> (w482:i32)
                  n382 = call "wait for SOMD ready.vi"("USB"=w482, "WaitTime"=15, "Max Loops"=750, "SLOT"=w481, "InpRefToOutput"=w480, "Stopp"=w479, "error in (no error)"=w474, "State Check Mask"=u16 51) -> ("error out"=w475:errorcluster)  [unwired: 3 in, 4 out]
                }
              }
            }
          }
          event "Combi Data": Value Change {
            n383 = event-data() -> ("OldVal"=w517:T4, "NewVal"=w518:T4)  [unwired: 1 in, 4 out]
            n384 = local read "Delay Data"() -> (w516:T3)
            n385 = local read "Burst Data"() -> (w515:T6)
            n386 = local read "SLOT"() -> (w514:i32)
            n387 = local read "USB"() -> (w513:i32)
            n388 = local read "Delayed Data"() -> (w511:T1)
            n389 = for {
              N: 8 -> [_]
              tunnel: w518 -> [w530] mode=indexing
              tunnel: w517 -> [w541] mode=indexing
              tunnel: w516 -> [w535] mode=indexing
              tunnel: w515 -> [w534] mode=indexing
              tunnel: w514 -> [w532]
              tunnel: w513 -> [w531]
              shift-right: [w522] -> _
              shift-left: _ -> [w521]
              tunnel: w511 -> [w520] mode=indexing
              tunnel: [w519] -> w510 mode=indexing
              i -> [w533]
              n390 = Unbundle By Name(w541) -> ("OutputCombi[i]"=w527:bool[], "MaskedCombi[i]"=w537:bool)
              n391 = Unbundle By Name(w530) -> ("OutputCombi[i]"=w528:bool[], "MaskedCombi[i]"=w529:bool)
              n392 = Boolean Array To Number(Boolean array=w527) -> (number=w538:u32)
              n393 = Boolean Array To Number(Boolean array=w528) -> (number=w525:u32)
              n394 = Equal To 0?(x=w525) -> (x = 0?=w526:bool)
              n395 = Select(t=w527, s=w526, f=w528) -> (s? t:f=w523:bool[])
              n396 = Bundle By Name(cluster=w530, "OutputCombi[i]"=w523, "MaskedCombi[i]"=w529) -> (w524:T2)
              n397 = Not Equal?(x=w538, y=w525) -> (x != y?=w539:bool)
              n398 = Not Equal?(x=w537, y=w529) -> (x != y?=w540:bool)
              n399 = Or(x=w539, y=w540) -> (x .or. y?=w536:bool)
              n400 = case shown="True" w536 {
                tunnel: w529 -> [_ w565]
                tunnel: w523 -> [_ w564]
                tunnel: w535 -> [_ w570]
                tunnel: w534 -> [_ w567]
                tunnel: w533 -> [_ w563]
                tunnel: w532 -> [_ w550]
                tunnel: w531 -> [_ w549]
                tunnel: w524 -> [_ w562]
                tunnel: [w543 w551] -> w522
                tunnel: w521 -> [w543 w561]
                tunnel: w520 -> [w542 w547]
                tunnel: [w542 w546] -> w519
                frame False {
                }
                frame True {
                  n401 = Unbundle By Name(w570) -> ("CoarseDelay[i]"=w569:dbl, "FineDelay[i]"=w568:u8)
                  n402 = Unbundle By Name(w567) -> ("Delayed[i]"=w566:bool)
                  n403 = case shown="0, Default" w563 {
                    tunnel: w562 -> [w571 w573 w575 w577 w579 w581 w583 w585]
                    frame 0, Default {
                      n404 = control-ref of="CombiDat 1"() -> (w572:refnum<vi>)
                      n405 = property class="Clust (strict)"(reference=w572, "Value"=w571) -> ()  [unwired: 1 in, 2 out]
                    }
                    frame 1 {
                      n406 = control-ref of="CombiDat 2"() -> (w574:refnum<vi>)
                      n407 = property class="Clust (strict)"(reference=w574, "Value"=w573) -> ()  [unwired: 1 in, 2 out]
                    }
                    frame 2 {
                      n408 = control-ref of="CombiDat 3"() -> (w576:refnum<vi>)
                      n409 = property class="Clust (strict)"(reference=w576, "Value"=w575) -> ()  [unwired: 1 in, 2 out]
                    }
                    frame 3 {
                      n410 = control-ref of="CombiDat 4"() -> (w578:refnum<vi>)
                      n411 = property class="Clust (strict)"(reference=w578, "Value"=w577) -> ()  [unwired: 1 in, 2 out]
                    }
                    frame 4 {
                      n412 = control-ref of="CombiDat 5"() -> (w580:refnum<vi>)
                      n413 = property class="Clust (strict)"(reference=w580, "Value"=w579) -> ()  [unwired: 1 in, 2 out]
                    }
                    frame 5 {
                      n414 = control-ref of="CombiDat 6"() -> (w582:refnum<vi>)
                      n415 = property class="Clust (strict)"(reference=w582, "Value"=w581) -> ()  [unwired: 1 in, 2 out]
                    }
                    frame 6 {
                      n416 = control-ref of="CombiDat 7"() -> (w584:refnum<vi>)
                      n417 = property class="Clust (strict)"(reference=w584, "Value"=w583) -> ()  [unwired: 1 in, 2 out]
                    }
                    frame 7 {
                      n418 = control-ref of="CombiDat 8"() -> (w586:refnum<vi>)
                      n419 = property class="Clust (strict)"(reference=w586, "Value"=w585) -> ()  [unwired: 1 in, 2 out]
                    }
                  }
                  n420 = To Unsigned Byte Integer(number=w563) -> (unsigned 8bit integer=w548:u8)
                  n421 = call "SOMD Set Sequencer Output Infos.vi"("DevIdx"=w549, "Output Combi"=w564, "Masked Combi"=w565, "SlotId"=w550, "Seq. Output Idx"=w548, "Delayed"=w566, "error in (no error)"=w561, "Coarse Delay"=w569, "Fine Delay"=w568) -> ("error out"=w553:errorcluster)  [unwired: 5 in, 1 out]
                  n422 = local read "Stopp"() -> (w557:bool)
                  n423 = local read "SLOT"() -> (w559:i32)
                  n424 = control-ref of="SOMD Status"() -> (w558:refnum<vi>)
                  n425 = local read "USB"() -> (w560:i32)
                  n426 = call "wait for SOMD ready.vi"("USB"=w560, "WaitTime"=15, "Max Loops"=750, "SLOT"=w559, "InpRefToOutput"=w558, "Stopp"=w557, "error in (no error)"=w553, "State Check Mask"=u16 51) -> ("error out"=w552:errorcluster)  [unwired: 3 in, 4 out]
                  n427 = call "SOMD Get Sequencer Output Infos.vi"("error in (no error)"=w552, "SeqOutputIdx"=w548, "SlotId"=w550, "DevIdx"=w549) -> ("error out"=w551:errorcluster, "Delayed"=w545:bool, "ForcedUndelayed"=w544:bool)  [unwired: 5 out]
                  n428 = Bundle By Name(cluster=w547, "ForcedUndelayed"=w544, "Delayed"=w545) -> (w546:cluster{"Delayed":bool, "ForcedUndelayed":bool})
                }
              }
            }
            n429 = local write "Delayed Data"(w510) -> ()
          }
          event "CombiDat 1", "CombiDat 2", "CombiDat 3", "CombiDat 4", "CombiDat 5", "CombiDat 6", "CombiDat 7", "CombiDat 8": Value Change {
            n430 = event-data() -> ()  [unwired: 1 in, 6 out]
            n431 = for {
              N: 8 -> [_]
              tunnel: [w589] -> w587 mode=indexing
              i -> [w590]
              n432 = case shown="7" w590 {
                tunnel: [w591 w592 w593 w594 w595 w596 w597 w598] -> w589
                frame 0, Default {
                  n433 = local read "CombiDat 1"() -> (w591:T2)
                }
                frame 1 {
                  n434 = local read "CombiDat 2"() -> (w592:T2)
                }
                frame 2 {
                  n435 = local read "CombiDat 3"() -> (w593:T2)
                }
                frame 3 {
                  n436 = local read "CombiDat 4"() -> (w594:T2)
                }
                frame 4 {
                  n437 = local read "CombiDat 5"() -> (w595:T2)
                }
                frame 5 {
                  n438 = local read "CombiDat 6"() -> (w596:T2)
                }
                frame 6 {
                  n439 = local read "CombiDat 7"() -> (w597:T2)
                }
                frame 7 {
                  n440 = local read "CombiDat 8"() -> (w598:T2)
                }
              }
            }
            n441 = local write "Combi Data"(w587) -> ()
          }
          event "DelayDat 1", "DelayDat 2", "DelayDat 3", "DelayDat 4", "DelayDat 5", "DelayDat 6", "DelayDat 7", "DelayDat 8": Value Change {
            n442 = event-data() -> ()  [unwired: 1 in, 6 out]
            n443 = for {
              N: 8 -> [_]
              tunnel: [w601] -> w599 mode=indexing
              i -> [w602]
              n444 = case shown="7" w602 {
                tunnel: [w603 w604 w605 w606 w607 w608 w609 w610] -> w601
                frame 0, Default {
                  n445 = local read "DelayDat 1"() -> (w603:cluster{"CoarseDelay[i]":dbl, "FineDelay[i]":u8})
                }
                frame 1 {
                  n446 = local read "DelayDat 2"() -> (w604:cluster{"CoarseDelay[i]":dbl, "FineDelay[i]":u8})
                }
                frame 2 {
                  n447 = local read "DelayDat 3"() -> (w605:cluster{"CoarseDelay[i]":dbl, "FineDelay[i]":u8})
                }
                frame 3 {
                  n448 = local read "DelayDat 4"() -> (w606:cluster{"CoarseDelay[i]":dbl, "FineDelay[i]":u8})
                }
                frame 4 {
                  n449 = local read "DelayDat 5"() -> (w607:cluster{"CoarseDelay[i]":dbl, "FineDelay[i]":u8})
                }
                frame 5 {
                  n450 = local read "DelayDat 6"() -> (w608:cluster{"CoarseDelay[i]":dbl, "FineDelay[i]":u8})
                }
                frame 6 {
                  n451 = local read "DelayDat 7"() -> (w609:cluster{"CoarseDelay[i]":dbl, "FineDelay[i]":u8})
                }
                frame 7 {
                  n452 = local read "DelayDat 8"() -> (w610:cluster{"CoarseDelay[i]":dbl, "FineDelay[i]":u8})
                }
              }
            }
            n453 = local write "Delay Data"(w599) -> ()
          }
          event "SyncNow": Value Change {
            n454 = event-data() -> ()  [unwired: 1 in, 6 out]
            n455 = local read "SLOT"() -> (w617:i32)
            n456 = control-ref of="SOMD Status"() -> (w615:refnum<vi>)
            n457 = local read "USB"() -> (w618:i32)
            n458 = call "SOMD Synchronize Now.vi"("SlotId"=w617, "DevIdx"=w618) -> ("error out"=w619:errorcluster)  [unwired: 1 in, 1 out]
            n459 = local read "Stopp"() -> (w616:bool)
            n460 = call "wait for SOMD ready.vi"("USB"=w618, "WaitTime"=35, "Max Loops"=1500, "SLOT"=w617, "InpRefToOutput"=w615, "Stopp"=w616, "error in (no error)"=w619, "State Check Mask"=u16 179) -> ("HW Ready to Run"=w613:bool, "error out"=w612:errorcluster)  [unwired: 3 in, 3 out]
            n461 = case shown="False" w613 {
              tunnel: w612 -> [w624 w638]
              tunnel: [w623 w636] -> w611
              frame False {
                w625 = 6
                n462 = property on="Burst Data" class="Arr (strict)"() -> ("Top"=w634:i32, "Left"=w633:i32, "Width"=w630:u32)  [unwired: 2 in, 2 out]
                n463 = property on="Sub Panel" class="SubPnl"() -> ("Width"=w626:u32, "Height"=w627:u32)  [unwired: 2 in, 2 out]
                n464 = Add(x=w626, y=w625) -> (x+y=w628:u32)
                n465 = Add(x=w625, y=w627) -> (x+y=w629:u32)
                n466 = Add(x=w630, y=w628) -> (x+y=w631:u32)
                n467 = property on="DisableBlend" class="Str"(error in=w624, "Top"=w634, "Left"=w633, "Width"=w631, "Height"=w629, "Visible"=TRUE) -> (error out=w623:errorcluster)  [unwired: 1 in, 1 out]
              }
              frame True {
                n468 = property on="USB" class="DigNum (strict)"() -> ("Top"=w641:i32, "Left"=w645:i32)  [unwired: 2 in, 2 out]
                n469 = Add(x=40, y=w641) -> (x+y=w642:i32)
                n470 = property on="DisableBlend" class="Str"(error in=w638, "Top"=w642, "Left"=w645, "Height"=u32 23, "Width"=u32 172 ("Size:Width"), "Visible"=TRUE) -> (error out=w635:errorcluster)  [unwired: 1 in, 1 out]
                n471 = local read "ExtTriggrd"() -> (w637:bool)
                n472 = property on="ExtTriggrd" class="Bool (strict)"(error in=w635, "Val(Sgnl)"=w637) -> (error out=w636:errorcluster)  [unwired: 1 in, 1 out]
              }
            }
            n473 = property on="SyncNow" class="Bool (strict)"(error in=w611, "Value"=FALSE ("SyncNow")) -> ()  [unwired: 1 in, 2 out]
          }
          event "Stopp": Value Change {
            n474 = event-data() -> ()  [unwired: 1 in, 6 out]
            n475 = property on="Stopp" class="Bool (strict)"("Val(Sgnl)"=TRUE ("Value (Signaling)")) -> ()  [unwired: 2 in, 2 out]
          }
          event Timeout {
            n476 = event-data() -> ()  [unwired: 1 in, 2 out]
          }
        }
        n477 = local read "Stopp"() -> (w194:bool)
      }
      n478 = node-c288(u32 750 ("y")) -> (w181:T7)  [unwired: 1 in]
      n479 = timed-loop {
        timing: w181 -> [_]
        timing-out: [_] -> w180
        stop <- w182 stop-if-true
        n480 = node-c288() -> ()  [unwired: 1 in, 1 out]
        n481 = local read "ExtTriggrd"() -> (w183:bool)
        n482 = case shown="True" w183 {
          frame False {
          }
          frame True {
            n483 = local read "SLOT"() -> (w186:i32)
            n484 = local read "USB"() -> (w187:i32)
            n485 = call "SOMD Get Trigger Sync Frequency.vi"("DevIdx"=w187, "SlotId"=w186) -> ("ExtFreq Stable"=w185:bool, "Trigger Sync Freq"=w184:u32)  [unwired: 1 in, 2 out]
            n486 = local write "Trigger Frequency"(w184) -> ()
            n487 = local write "FreqStable"(w185) -> ()
          }
        }
        n488 = local read "Stopp"() -> (w182:bool)
        n489 = node-c288() -> ()  [unwired: 1 out]
      }
      n490 = node-c288(w180) -> ()
    }
    frame #4 {
      w647 = TRUE
      n491 = local write "Stopp"(FALSE ("Stopp")) -> ()
      n492 = property on="TriggerLevel [mV]" class="DigNum (strict)"("Visible"=w647) -> ()  [unwired: 2 in, 2 out]
      n493 = property on="Trigger Frequency" class="DigNum (strict)"("Visible"=w647) -> ()  [unwired: 2 in, 2 out]
      n494 = property on="Synchronize" class="Bool (strict)"("Visible"=w647) -> ()  [unwired: 2 in, 2 out]
      n495 = property on="FreqStable" class="Bool (strict)"("Visible"=w647) -> ()  [unwired: 2 in, 2 out]
      n496 = property on="SyncNow" class="Bool (strict)"("Visible"=w647) -> ()  [unwired: 2 in, 2 out]
    }
  }
